vi "ramp.vi"(4 "State":i16, 5 "Time":dbl format="%.2f", 6 "Sensor Values":dbl[](array[numeric]), 7 "Set Points":dbl[](array[numeric])) -> (0 "required data":T1={"Set Point names"=["initial value", "final value", "ramp time"], "required number of setpoints"=3, "required number of sensors"=1, "Sensor names"=["time in state"]}, 3 "output value":dbl)   [LabVIEW 2012]
panel:
  # "Enter the correct information for this control code in the required data structure below. Then make the current value default by right clicking on the border of the data structure. Select \"data operations\" and then select \"make current value default\". These values will be displayed by process controller."
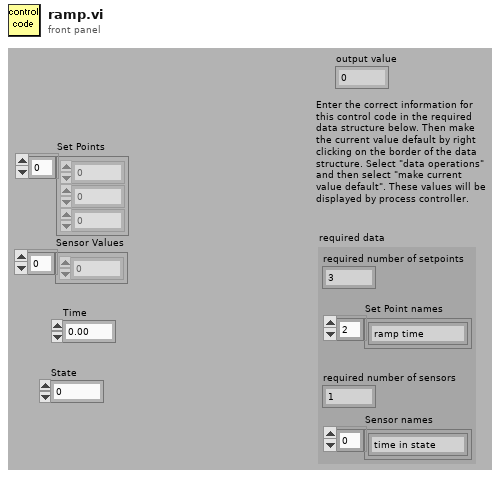
[diagram p1: front panel]
types:
  T1 = cluster{"Set Point names":string[], "required number of setpoints":u8, "required number of sensors":u8, "Sensor names":string[]}
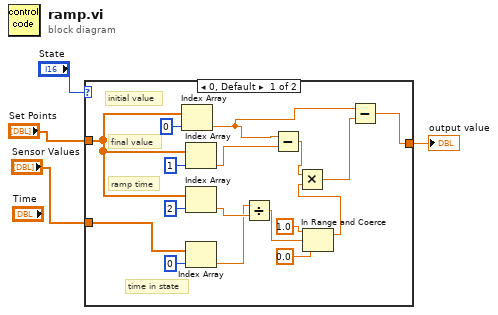
[diagram p0: block diagram]
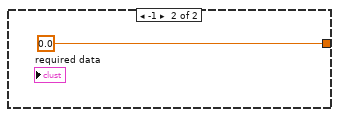
[diagram p2: hidden frame]
diagram:
  n1 = case shown="0, Default" "State" {
    tunnel: [w12 0.0 ("fraction on")] -> w3
    tunnel: "Set Points" -> [w18 _]
    tunnel: "Sensor Values" -> [w6 _]
    frame 0, Default {
      # "time in state"
      # "ramp time"
      # "final value"
      # "initial value"
      n2 = Index Array(array=w18, index=0) -> (element=w14:dbl)
      n3 = Index Array(array=w18, index=1) -> (element=w17:dbl)
      n4 = Index Array(array=w18, index=2) -> (element=w16:dbl)
      n5 = Index Array(array=w6, index=0) -> (element=w5:dbl)
      n6 = Divide(x=w5, y=w16) -> (x/y=w9:dbl)
      n7 = Subtract(x=w14, y=w17) -> (x-y=w15:dbl)
      n8 = In Range and Coerce(upper limit=1.0, x=w9, lower limit=0.0) -> (coerced(x)=w8:dbl)  [unwired: 1 out]
      n9 = Multiply(x=w15, y=w8) -> (x*y=w13:dbl)
      n10 = Subtract(x=w14, y=w13) -> (x-y=w12:dbl)
    }
    frame -1 {
    }
  }
  "output value" <- w3
